vi "FTW-Test-JSON-Stress.vi"() -> (0 "Test Result":errorcluster)   [LabVIEW 2014]
uses:
  src/core/error/FTW-ERR-Assert-DeveloperError.vi
  src/core/error/FTW-ERR-ThrowError.vi
  src/core/error/FTW-ERR-CallChain.vi
  src/core/string/FTW-STR-ReplaceWhitespace.vi
panel:
  out "Serialized JSON":string[](array[string])
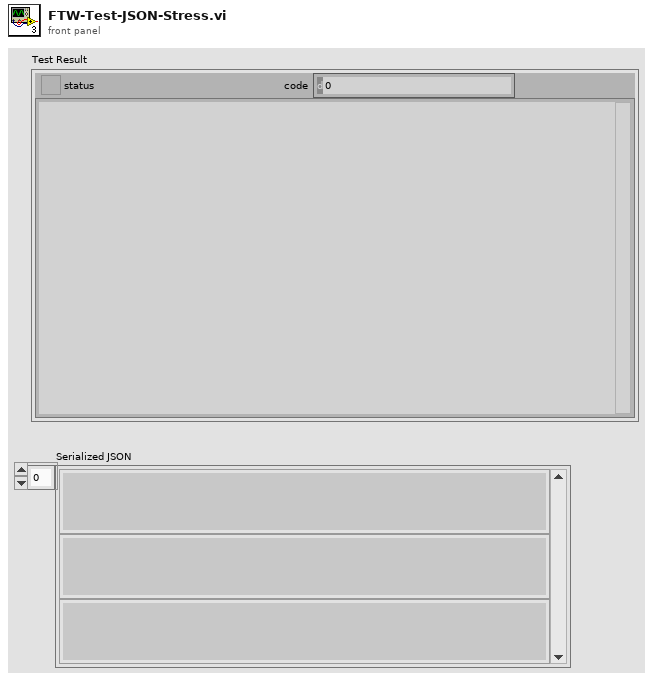
[diagram p1: front panel]
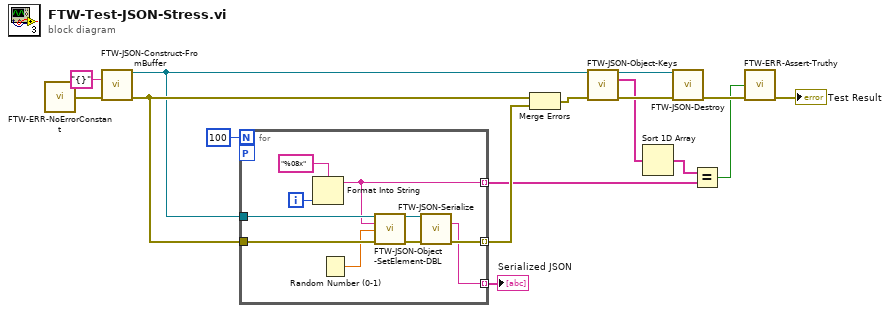
[diagram p0: block diagram]
diagram:
  n1 = call "FTW-ERR-NoErrorConstant.vi"() -> ("no error"=w4:errorcluster)
  n2 = call "FTW-JSON-Construct-FromBuffer.vi"("JSON String (UTF-8)"="{}", "error in"=w4) -> ("JSON Object"=w12:refnum<data-value>, "error out"=w13:errorcluster)  [unwired: 12 in]
  n3 = for {
    N: 100 -> [_]
    tunnel: [w22] -> w1 mode=indexing
    workers-P: _ -> [_]
    tunnel: w13 -> [w25]
    tunnel: [w24] -> w14 mode=indexing
    tunnel: w12 -> [w26]
    tunnel: [w17] -> w10 mode=indexing
    i -> [w18]
    n4 = Format Into String(format string="%08x", w18) -> (resulting string=w17:string)  [unwired: 2 in, 1 out]
    n5 = Random Number (0-1)() -> (number: 0 to 1=w23:dbl)
    n6 = call "FTW-JSON-Object-SetElement-DBL.vi"("JSON Object"=w26, "Key"=w17, "Value"=w23, "error in"=w25) -> ("JSON Object out"=w21:refnum<data-value>, "error out"=w20:errorcluster)  [unwired: 10 in]
    n7 = call "FTW-JSON-Serialize.vi"("JSON Object"=w21, "error in"=w20) -> ("JSON String (UTF-8)"=w22:string, "error out"=w24:errorcluster)  [unwired: 11 in, 1 out]
  }
  "Serialized JSON" <- w1
  n8 = Merge Errors(w13, w14) -> (w11:errorcluster)
  n9 = call "FTW-JSON-Object-Keys.vi"("JSON Object"=w12, "error in"=w11) -> ("JSON Object out"=w9:refnum<data-value>, "Keys"=w3:string[], "error out"=w8:errorcluster)  [unwired: 10 in, 1 out]
  n10 = Sort 1D Array(array=w3) -> (sorted array=w2:string[])
  n11 = call "FTW-JSON-Destroy.vi"("JSON Object"=w9, "error in"=w8) -> ("error out"=w7:errorcluster)  [unwired: 13 in]
  n12 = Equal?(x=w2, y=w10) -> (x = y?=w6:bool)
  n13 = call "FTW-ERR-Assert-Truthy.vi"("Expected Truthy"=w6, "error in"=w7) -> ("error out"=→"Test Result":errorcluster)  [unwired: 13 in]
